vi "DiffKinematics_toTwist2d.vi"(9 "Right Distance M":dbl, 10 "Left Distance M":dbl, 11 "DIFF_DRIVE_KINEMATICS":T1 {"TrackWidth_Meters" format="%20.4f"}) -> (3 "Twist2d":T2)   [LabVIEW 2019, in "Trajectory_Library.lvlib"]
doc: "Returns left and right component velocities from a chassis speed using inverse kinematics.\n\nParameters:\n - DiffDriveKinematics - This differential drive kinematics data structure\n - chassisSpeeds - The linear and angular (dx and dtheta) components that represent the chassis' speed.\n\nReturns:\n - LeftVelocity - Left wheel velocity (meters/sec )\n - RightVelocity - Right wheel velocity (meters/sec)"
uses:
  TypeDef/DIFF_DRIVE_KINEMATICS.ctl
  Trajectory_Library.lvlib
  TypeDef/TWIST2D.ctl
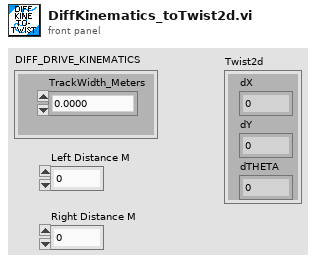
[diagram p1: front panel]
types:
  T1 = typedef "Trajectory_Library.lvlib/DIFF_DRIVE_KINEMATICS.ctl" = cluster{"TrackWidth_Meters":dbl}
  T2 = typedef "Trajectory_Library.lvlib/TWIST2D.ctl" = cluster{"dX":dbl, "dY":dbl, "dTHETA":dbl}
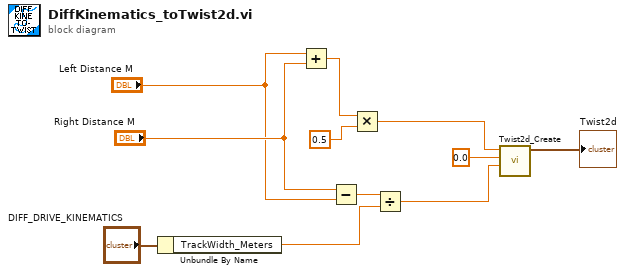
[diagram p0: block diagram]
diagram:
  n1 = Unbundle By Name("DIFF_DRIVE_KINEMATICS") -> ("TrackWidth_Meters"=w3:dbl)
  n2 = Add(x="Left Distance M", y="Right Distance M") -> (x+y=w9:dbl)
  n3 = Subtract(x="Right Distance M", y="Left Distance M") -> (x-y=w4:dbl)
  n4 = Multiply(x=w9, y=0.5) -> (x*y=w8:dbl)
  n5 = Divide(x=w4, y=w3) -> (x/y=w2:dbl)
  n6 = call "Twist2d_Create.vi"("dTHETA"=w2, "dY"=0.0, "dX"=w8) -> ("TWIST"=→"Twist2d":T2)  [unwired: 8 in]
